vi "Select.vi"(8 "error in (no error)":errorcluster, 10 "State":string(combo), 11 "Reference Cluster":T1) -> (0 "error out":errorcluster, 2 "Count error?":bool, 3 "Confirmed?":bool)   [LabVIEW 2019, in "ZenGage v3.0 UI.lvclass"]
uses:
  ZenGage v3.0 UI.lvclass
panel:
  out "Verification":bool
  in  "Change":bool
  in  "Confirm":bool
  in  "OK Button":bool
  in  "Reset Button":bool
  in  "Total Count":string
  in  "Reel Count":string
  in  "Operator ID":string
  in  "Part Name":string(combo)
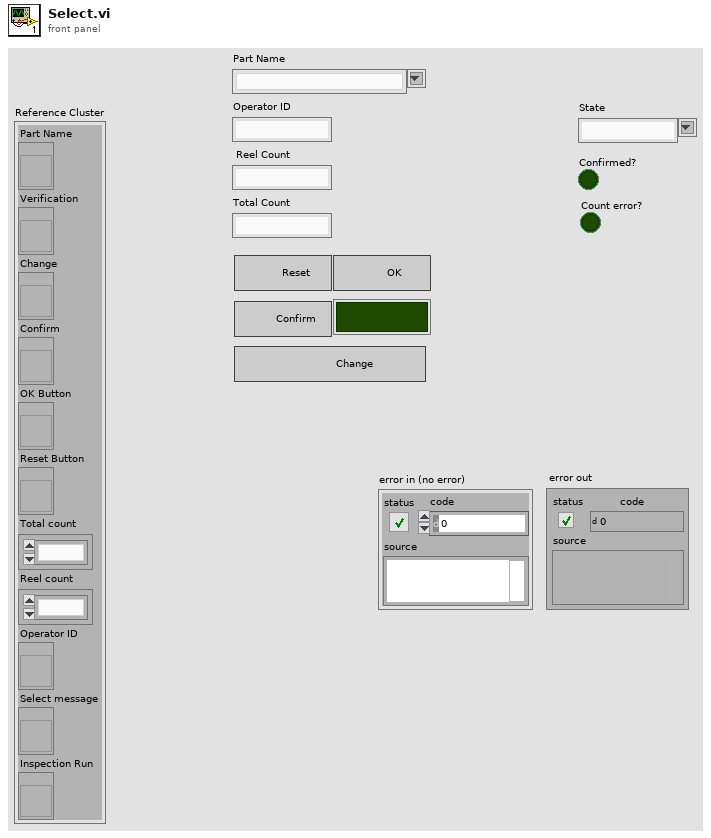
[diagram p1: front panel]
types:
  T1 = cluster{"Part Name":refnum<vi>, "Verification":refnum<vi>, "Change":refnum<vi>, "Confirm":refnum<vi>, "OK Button":refnum<vi>, "Reset Button":refnum<vi>, "Total count":refnum<vi>, "Reel count":refnum<vi>, "Operator ID":refnum<vi>, "Select message":refnum<vi>, "Inspection Run":refnum<vi>}
  T2 = enum8{"Enabled", "Disabled", "Disabled and Grayed Out"}
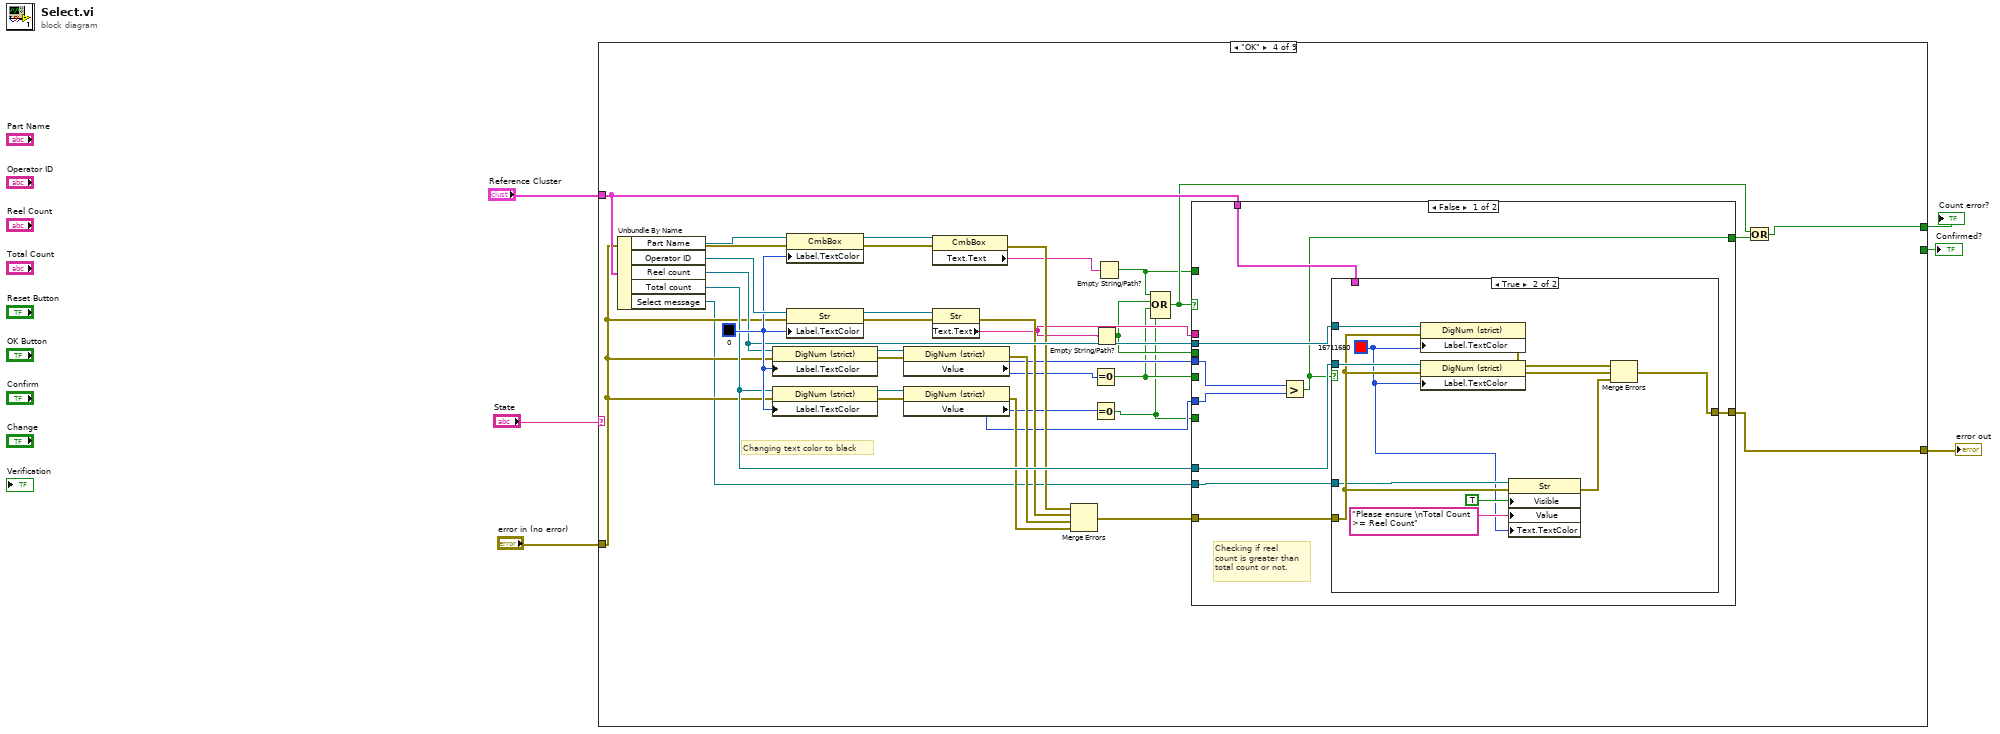
[diagram p0: block diagram]
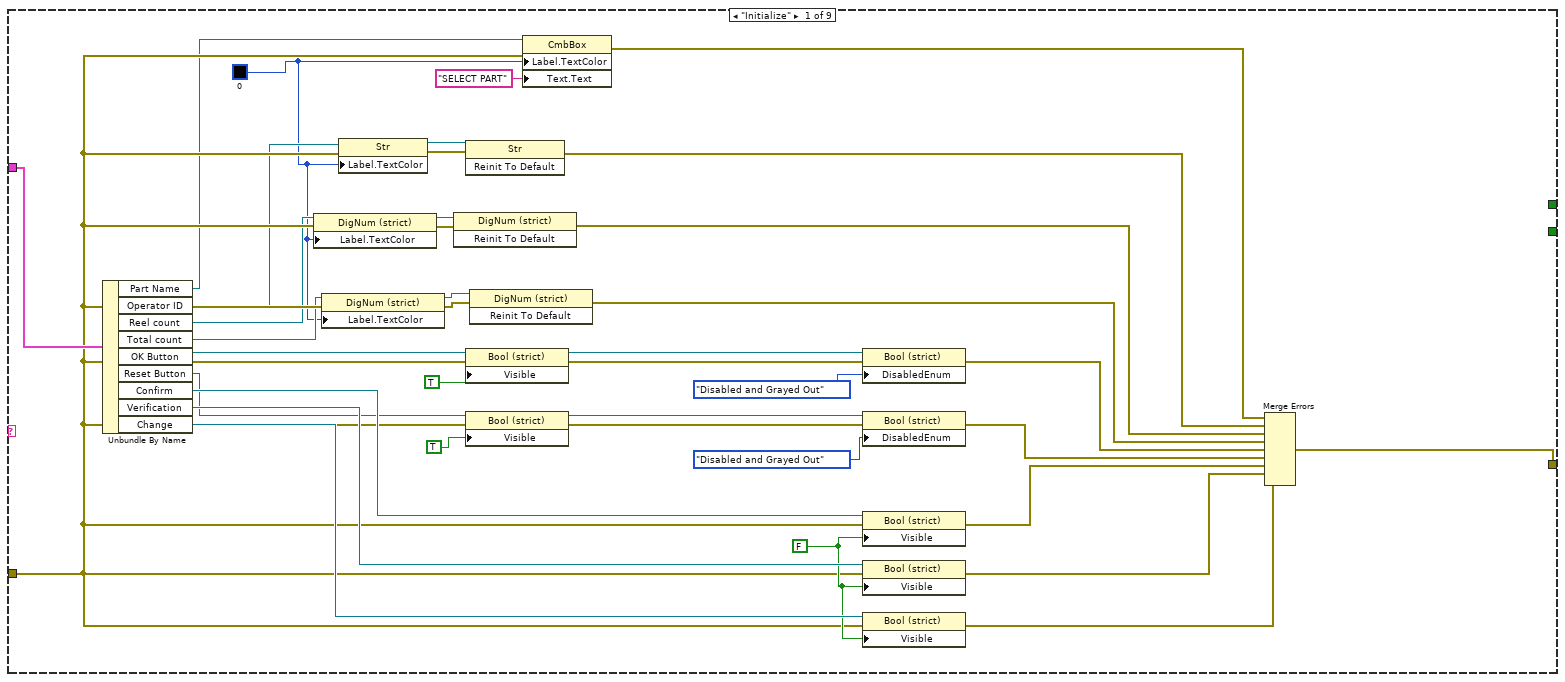
[diagram p2: hidden frame]
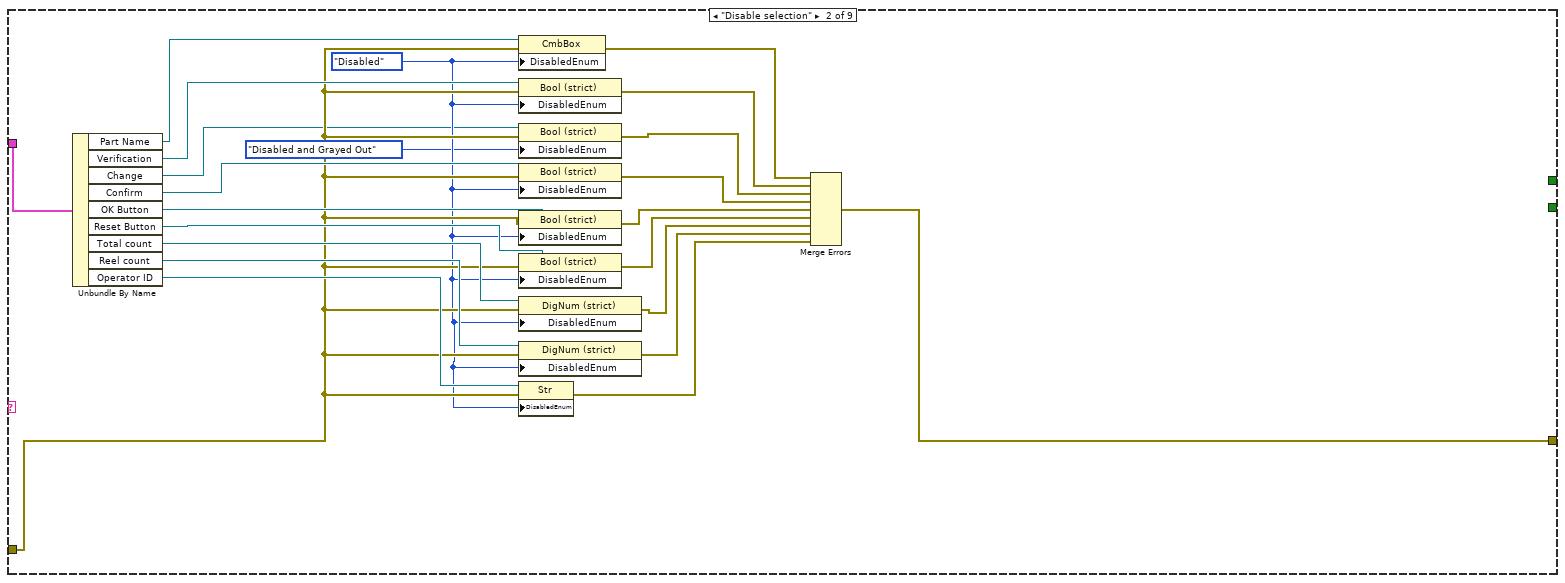
[diagram p3: hidden frame]
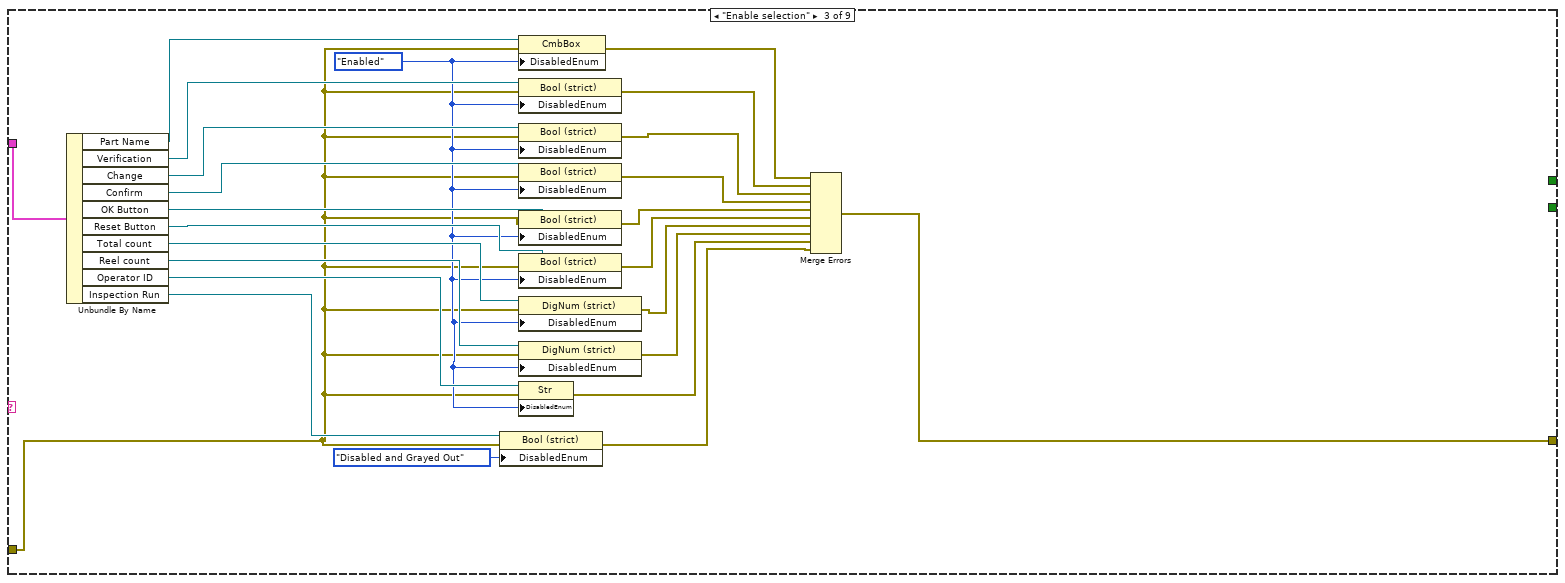
[diagram p4: hidden frame]
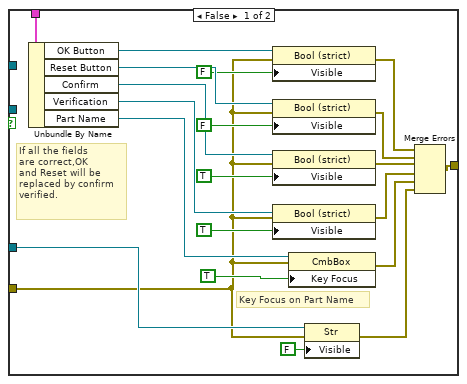
[diagram p5: hidden frame]
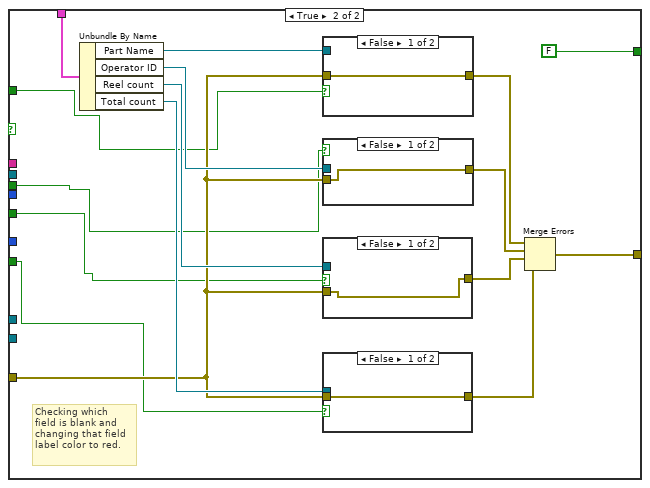
[diagram p6: hidden frame]
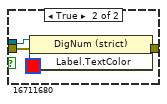
[diagram p7: hidden frame]
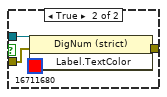
[diagram p8: hidden frame]
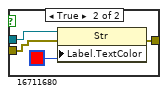
[diagram p9: hidden frame]
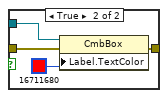
[diagram p10: hidden frame]
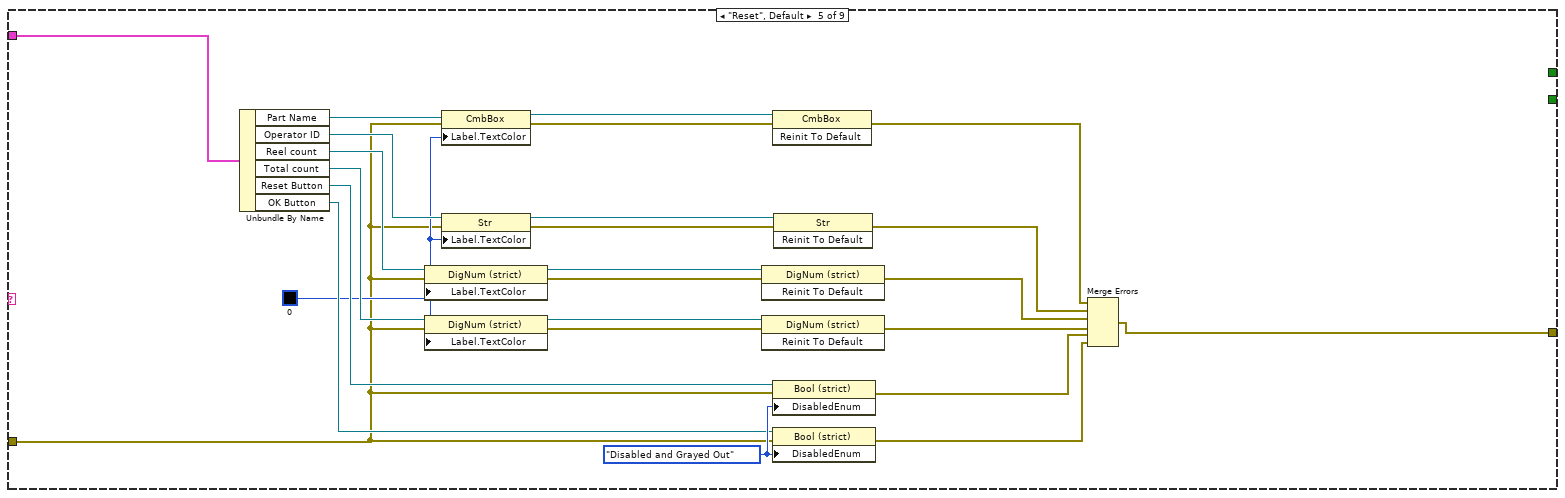
[diagram p11: hidden frame]
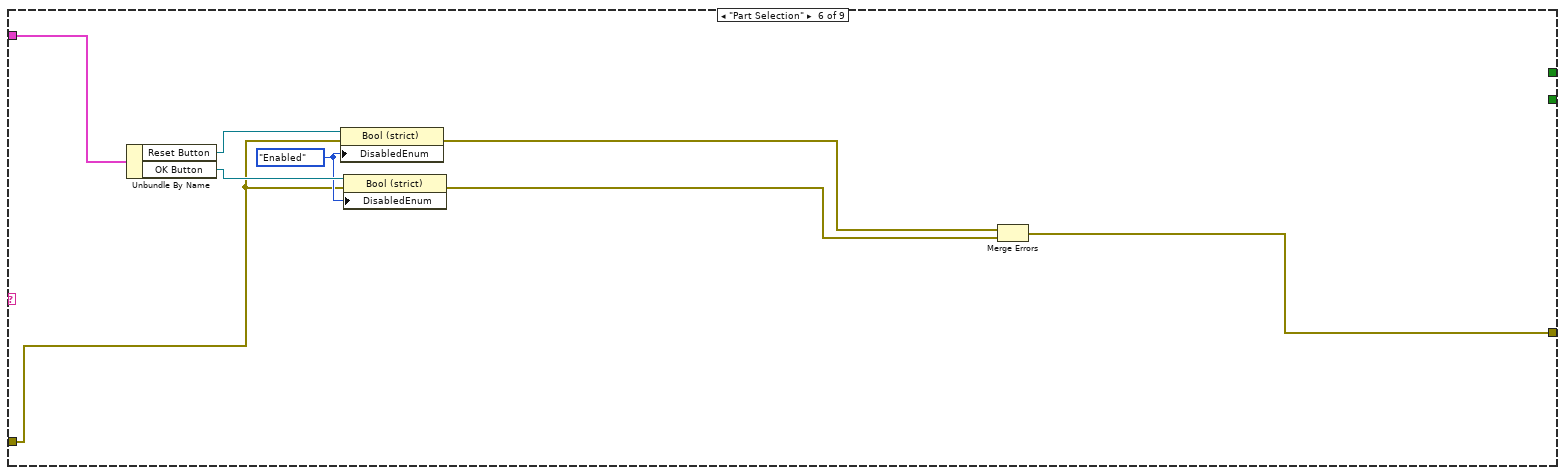
[diagram p12: hidden frame]
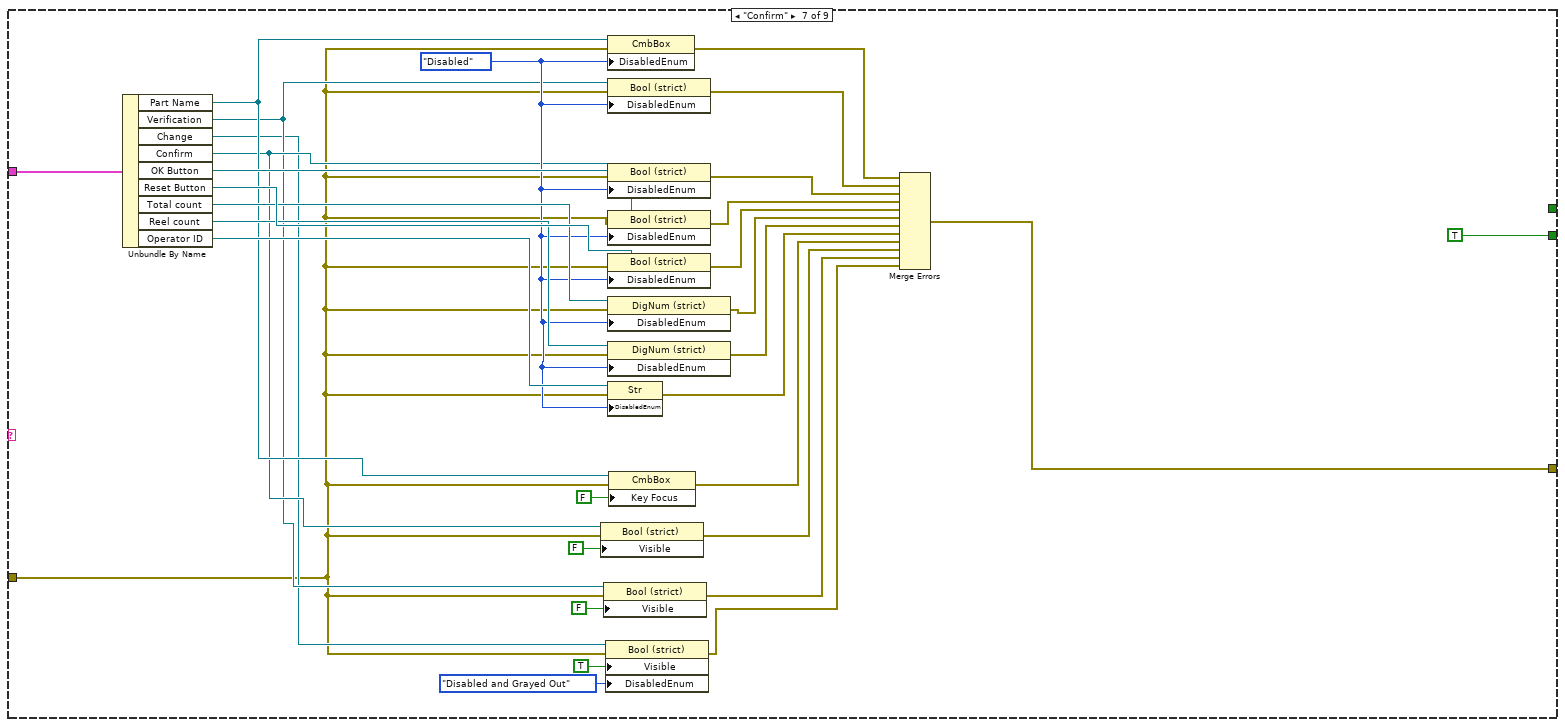
[diagram p13: hidden frame]
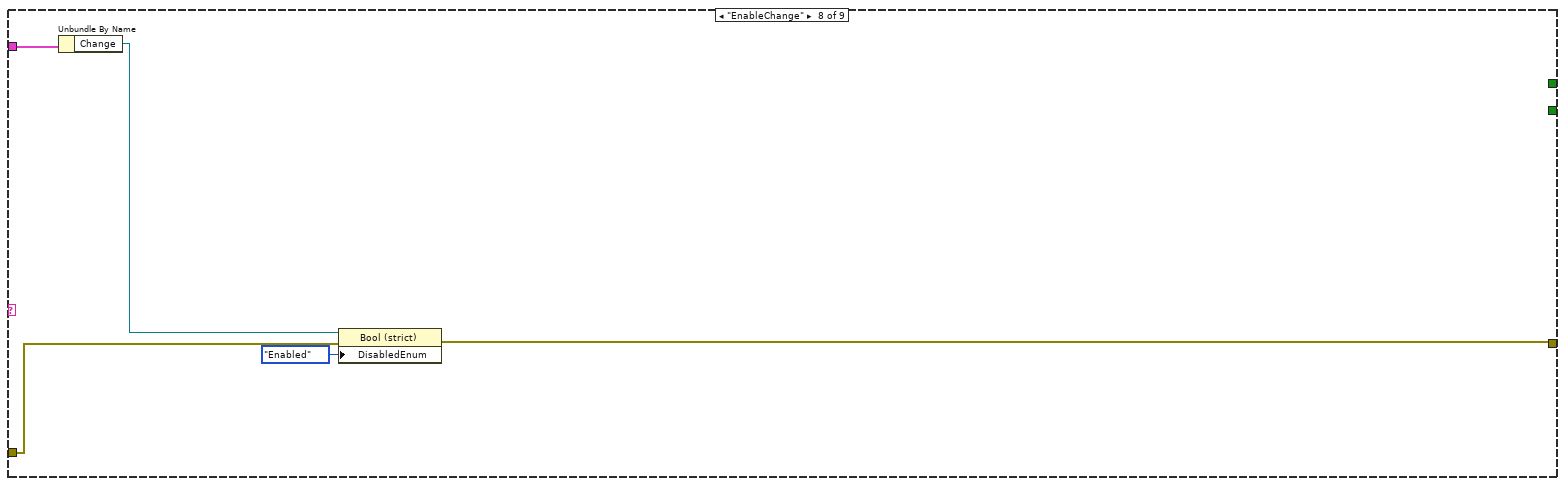
[diagram p14: hidden frame]
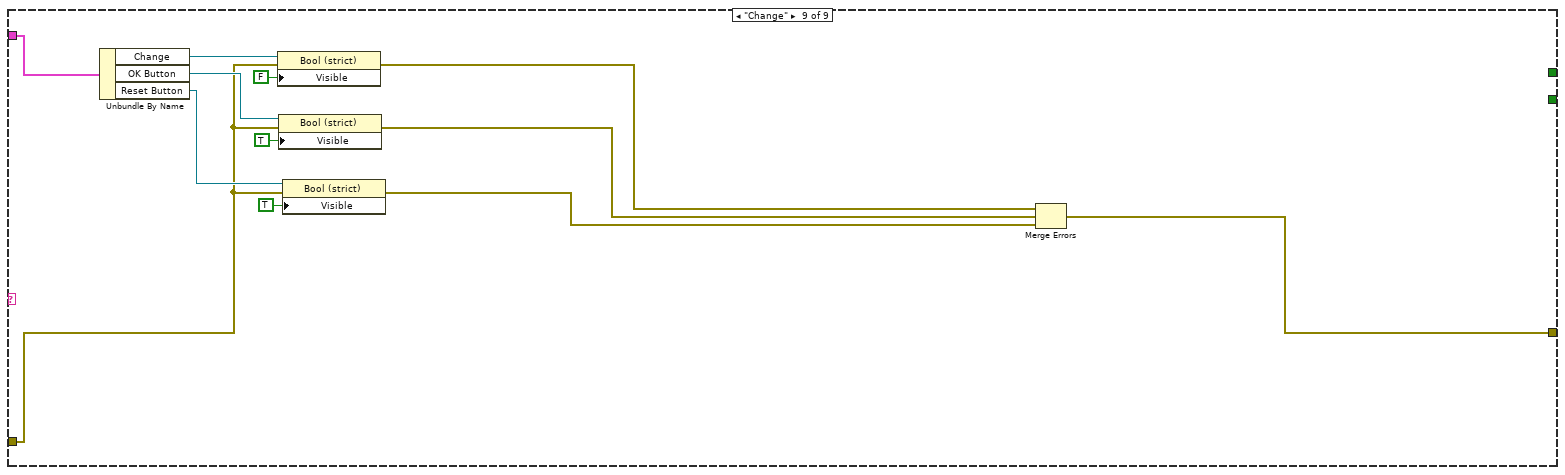
[diagram p15: hidden frame]
diagram:
  n1 = case shown="\"OK\"" "State" {
    tunnel: "Reference Cluster" -> [w42 w67 w92 w116 w219 w232 w243 w271 w283]
    tunnel: "error in (no error)" -> [w18 w49 w69 w115 w204 w228 w242 w270 w276]
    tunnel: [w32 w48 w73 w105 w203 w229 w237 w269 w272] -> w3
    tunnel: [_ _ _ _ _ _ TRUE _ _] -> w2
    tunnel: [_ _ _ w98 _ _ _ _ _] -> w1
    frame "Initialize" {
      w9 = u32 0
      w38 = FALSE ("Visible")
      n2 = Unbundle By Name(w42) -> ("Part Name"=w10:refnum<vi>, "Operator ID"=w16:refnum<vi>, "Reel count"=w14:refnum<vi>, "Total count"=w12:refnum<vi>, "OK Button"=w26:refnum<vi>, "Reset Button"=w24:refnum<vi>, "Confirm"=w41:refnum<vi>, "Verification"=w40:refnum<vi>, "Change"=w39:refnum<vi>)
      n3 = property class="DigNum (strict)"(reference=w14, error in=w18, "Label.TextColor"=w9) -> (reference out=w13:refnum<vi>, error out=w19:errorcluster)
      n4 = property class="DigNum (strict)"(reference=w12, error in=w18, "Label.TextColor"=w9) -> (reference out=w11:refnum<vi>, error out=w17:errorcluster)
      n5 = property class="Str"(reference=w16, error in=w18, "Label.TextColor"=w9) -> (reference out=w15:refnum<vi>, error out=w20:errorcluster)
      n6 = invoke class="DigNum (strict)" method="Reinit To Default"(reference=w13, error in=w19) -> (error out=w22:errorcluster)  [unwired: 1 in, 2 out]
      n7 = invoke class="Str" method="Reinit To Default"(reference=w15, error in=w20) -> (error out=w23:errorcluster)  [unwired: 1 in, 2 out]
      n8 = property class="Bool (strict)"(reference=w26, error in=w18, "Visible"=TRUE ("Value")) -> (reference out=w27:refnum<vi>, error out=w28:errorcluster)
      n9 = property class="Bool (strict)"(reference=w24, error in=w18, "Visible"=TRUE) -> (reference out=w31:refnum<vi>, error out=w30:errorcluster)
      n10 = invoke class="DigNum (strict)" method="Reinit To Default"(reference=w11, error in=w17) -> (error out=w21:errorcluster)  [unwired: 1 in, 2 out]
      n11 = property class="CmbBox"(reference=w10, error in=w18, "Label.TextColor"=w9, "Text.Text"="SELECT PART") -> (error out=w8:errorcluster)  [unwired: 1 out]
      n12 = property class="Bool (strict)"(reference=w27, error in=w28, "DisabledEnum"=T2."Disabled and Grayed Out" ("Disabled")) -> (error out=w37:errorcluster)  [unwired: 1 out]
      n13 = property class="Bool (strict)"(reference=w31, error in=w30, "DisabledEnum"=T2."Disabled and Grayed Out" ("Disabled")) -> (error out=w36:errorcluster)  [unwired: 1 out]
      n14 = property class="Bool (strict)"(reference=w41, error in=w18, "Visible"=w38) -> (error out=w35:errorcluster)  [unwired: 1 out]
      n15 = property class="Bool (strict)"(reference=w40, error in=w18, "Visible"=w38) -> (error out=w34:errorcluster)  [unwired: 1 out]
      n16 = property class="Bool (strict)"(reference=w39, error in=w18, "Visible"=w38) -> (error out=w33:errorcluster)  [unwired: 1 out]
      n17 = Merge Errors(w8, w23, w22, w21, w37, w36, w35, w34, w33) -> (w32:errorcluster)
    }
    frame "Disable selection" {
      w47 = T2."Disabled" ("Disabled")
      n18 = Unbundle By Name(w67) -> ("Part Name"=w66:refnum<vi>, "Verification"=w65:refnum<vi>, "Change"=w45:refnum<vi>, "Confirm"=w64:refnum<vi>, "OK Button"=w63:refnum<vi>, "Reset Button"=w62:refnum<vi>, "Total count"=w61:refnum<vi>, "Reel count"=w60:refnum<vi>, "Operator ID"=w59:refnum<vi>)
      n19 = property class="CmbBox"(reference=w66, error in=w49, "DisabledEnum"=w47) -> (error out=w58:errorcluster)  [unwired: 1 out]
      n20 = property class="Bool (strict)"(reference=w65, error in=w49, "DisabledEnum"=w47) -> (error out=w57:errorcluster)  [unwired: 1 out]
      n21 = property class="Bool (strict)"(reference=w45, error in=w49, "DisabledEnum"=T2."Disabled and Grayed Out" ("Disabled")) -> (error out=w56:errorcluster)  [unwired: 1 out]
      n22 = property class="Bool (strict)"(reference=w64, error in=w49, "DisabledEnum"=w47) -> (error out=w55:errorcluster)  [unwired: 1 out]
      n23 = property class="Bool (strict)"(reference=w63, error in=w49, "DisabledEnum"=w47) -> (error out=w54:errorcluster)  [unwired: 1 out]
      n24 = property class="Bool (strict)"(reference=w62, error in=w49, "DisabledEnum"=w47) -> (error out=w53:errorcluster)  [unwired: 1 out]
      n25 = property class="DigNum (strict)"(reference=w61, error in=w49, "DisabledEnum"=w47) -> (error out=w52:errorcluster)  [unwired: 1 out]
      n26 = property class="DigNum (strict)"(reference=w60, error in=w49, "DisabledEnum"=w47) -> (error out=w51:errorcluster)  [unwired: 1 out]
      n27 = property class="Str"(reference=w59, error in=w49, "DisabledEnum"=w47) -> (error out=w50:errorcluster)  [unwired: 1 out]
      n28 = Merge Errors(w58, w57, w56, w55, w54, w53, w52, w51, w50) -> (w48:errorcluster)
    }
    frame "Enable selection" {
      w72 = T2."Enabled" ("Disabled")
      n29 = Unbundle By Name(w92) -> ("Part Name"=w91:refnum<vi>, "Verification"=w90:refnum<vi>, "Change"=w89:refnum<vi>, "Confirm"=w88:refnum<vi>, "OK Button"=w87:refnum<vi>, "Reset Button"=w86:refnum<vi>, "Total count"=w85:refnum<vi>, "Reel count"=w84:refnum<vi>, "Operator ID"=w83:refnum<vi>, "Inspection Run"=w71:refnum<vi>)
      n30 = property class="Bool (strict)"(reference=w71, error in=w69, "DisabledEnum"=T2."Disabled and Grayed Out" ("Disabled")) -> (error out=w68:errorcluster)  [unwired: 1 out]
      n31 = property class="CmbBox"(reference=w91, error in=w69, "DisabledEnum"=w72) -> (error out=w82:errorcluster)  [unwired: 1 out]
      n32 = property class="Bool (strict)"(reference=w90, error in=w69, "DisabledEnum"=w72) -> (error out=w81:errorcluster)  [unwired: 1 out]
      n33 = property class="Bool (strict)"(reference=w89, error in=w69, "DisabledEnum"=w72) -> (error out=w80:errorcluster)  [unwired: 1 out]
      n34 = property class="Bool (strict)"(reference=w88, error in=w69, "DisabledEnum"=w72) -> (error out=w79:errorcluster)  [unwired: 1 out]
      n35 = property class="Bool (strict)"(reference=w87, error in=w69, "DisabledEnum"=w72) -> (error out=w78:errorcluster)  [unwired: 1 out]
      n36 = property class="Bool (strict)"(reference=w86, error in=w69, "DisabledEnum"=w72) -> (error out=w77:errorcluster)  [unwired: 1 out]
      n37 = property class="DigNum (strict)"(reference=w85, error in=w69, "DisabledEnum"=w72) -> (error out=w76:errorcluster)  [unwired: 1 out]
      n38 = property class="DigNum (strict)"(reference=w84, error in=w69, "DisabledEnum"=w72) -> (error out=w75:errorcluster)  [unwired: 1 out]
      n39 = property class="Str"(reference=w83, error in=w69, "DisabledEnum"=w72) -> (error out=w74:errorcluster)  [unwired: 1 out]
      n40 = Merge Errors(w82, w81, w80, w79, w78, w77, w76, w75, w74, w68) -> (w73:errorcluster)
    }
    frame "OK" {
      w119 = u32 0
      # "Changing text color to black"
      n41 = Unbundle By Name(w116) -> ("Part Name"=w125:refnum<vi>, "Operator ID"=w124:refnum<vi>, "Reel count"=w118:refnum<vi>, "Total count"=w117:refnum<vi>, "Select message"=w93:refnum<vi>)
      n42 = property class="DigNum (strict)"(reference=w118, error in=w115, "Label.TextColor"=w119) -> (reference out=w121:refnum<vi>, error out=w112:errorcluster)
      n43 = property class="DigNum (strict)"(reference=w117, error in=w115, "Label.TextColor"=w119) -> (reference out=w120:refnum<vi>, error out=w111:errorcluster)
      n44 = property class="CmbBox"(reference=w125, error in=w115, "Label.TextColor"=w119) -> (reference out=w123:refnum<vi>, error out=w114:errorcluster)
      n45 = property class="Str"(reference=w124, error in=w115, "Label.TextColor"=w119) -> (reference out=w122:refnum<vi>, error out=w113:errorcluster)
      n46 = property class="DigNum (strict)"(reference=w121, error in=w112) -> (error out=w108:errorcluster, "Value"=w102:u64)  [unwired: 1 out]
      n47 = property class="DigNum (strict)"(reference=w120, error in=w111) -> (error out=w107:errorcluster, "Value"=w101:u64)  [unwired: 1 out]
      n48 = property class="CmbBox"(reference=w123, error in=w114) -> (error out=w110:errorcluster, "Text.Text"=w104:string)  [unwired: 1 out]
      n49 = property class="Str"(reference=w122, error in=w113) -> (error out=w109:errorcluster, "Text.Text"=w103:string)  [unwired: 1 out]
      n50 = Merge Errors(w110, w109, w108, w107) -> (w106:errorcluster)
      n51 = Equal To 0?(x=w102) -> (x = 0?=w95:bool)
      n52 = Equal To 0?(x=w101) -> (x = 0?=w94:bool)
      n53 = Empty String/Path?(string/path=w103) -> (empty?=w96:bool)
      n54 = Empty String/Path?(string/path=w104) -> (empty?=w97:bool)
      n55 = Compound Arithmetic op=OR(w97, w96, w95, w94) -> (w99:bool)
      n56 = case shown="False" w99 {
        tunnel: w102 -> [w134 _]
        tunnel: w101 -> [w133 _]
        tunnel: w118 -> [w132 _]
        tunnel: w117 -> [w131 _]
        tunnel: w103 -> [_ _]
        tunnel: w116 -> [w130 w182]
        tunnel: w106 -> [w129 w177]
        tunnel: [w128 w172] -> w105
        tunnel: [w127 FALSE] -> w100
        tunnel: w97 -> [_ w170]
        tunnel: w96 -> [_ w169]
        tunnel: w95 -> [_ w168]
        tunnel: w94 -> [_ w167]
        tunnel: w93 -> [w126 _]
        frame False {
          # "Checking if reel\ncount is greater than\ntotal count or not."
          n57 = Greater?(x=w134, y=w133) -> (0:w127:bool)
          n58 = case shown="True" w127 {
            tunnel: w132 -> [_ w165]
            tunnel: w131 -> [_ w166]
            tunnel: w130 -> [w155 _]
            tunnel: w129 -> [w136 w161]
            tunnel: [w139 w162] -> w128
            tunnel: w126 -> [w138 w159]
            frame False {
              # "Key Focus on Part Name"
              # "If all the fields \nare correct,OK\nand Reset will be \nreplaced by confirm\nverified."
              n59 = Unbundle By Name(w155) -> ("OK Button"=w151:refnum<vi>, "Reset Button"=w152:refnum<vi>, "Confirm"=w153:refnum<vi>, "Verification"=w154:refnum<vi>, "Part Name"=w146:refnum<vi>)
              n60 = property class="Bool (strict)"(reference=w151, error in=w136, "Visible"=FALSE) -> (error out=w144:errorcluster)  [unwired: 1 out]
              n61 = property class="Bool (strict)"(reference=w152, error in=w136, "Visible"=FALSE) -> (error out=w143:errorcluster)  [unwired: 1 out]
              n62 = property class="Bool (strict)"(reference=w153, error in=w136, "Visible"=TRUE) -> (error out=w142:errorcluster)  [unwired: 1 out]
              n63 = property class="Bool (strict)"(reference=w154, error in=w136, "Visible"=TRUE) -> (error out=w141:errorcluster)  [unwired: 1 out]
              n64 = property class="CmbBox"(reference=w146, error in=w136, "Key Focus"=TRUE ("Visible")) -> (error out=w140:errorcluster)  [unwired: 1 out]
              n65 = property class="Str"(reference=w138, error in=w136, "Visible"=FALSE) -> (error out=w135:errorcluster)  [unwired: 1 out]
              n66 = Merge Errors(w144, w143, w142, w141, w140, w135) -> (w139:errorcluster)
            }
            frame True {
              w156 = u32 16711680
              n67 = property class="DigNum (strict)"(reference=w165, error in=w161, "Label.TextColor"=w156) -> (error out=w164:errorcluster)  [unwired: 1 out]
              n68 = property class="DigNum (strict)"(reference=w166, error in=w161, "Label.TextColor"=w156) -> (error out=w163:errorcluster)  [unwired: 1 out]
              n69 = property class="Str"(reference=w159, error in=w161, "Visible"=TRUE, "Value"="Please ensure \nTotal Count >= Reel Count", "Text.TextColor"=w156) -> (error out=w160:errorcluster)  [unwired: 1 out]
              n70 = Merge Errors(w164, w163, w160) -> (w162:errorcluster)
            }
          }
        }
        frame True {
          # "Checking which \nfield is blank and\nchanging that field\nlabel color to red."
          n71 = Unbundle By Name(w182) -> ("Part Name"=w181:refnum<vi>, "Operator ID"=w180:refnum<vi>, "Reel count"=w179:refnum<vi>, "Total count"=w178:refnum<vi>)
          n72 = case shown="False" w170 {
            tunnel: w181 -> [_ w201]
            tunnel: w177 -> [w198 w200]
            tunnel: [w198 w199] -> w176
            frame False {
            }
            frame True {
              n73 = property class="CmbBox"(reference=w201, error in=w200, "Label.TextColor"=u32 16711680) -> (error out=w199:errorcluster)  [unwired: 1 out]
            }
          }
          n74 = case shown="False" w169 {
            tunnel: w180 -> [_ w196]
            tunnel: w177 -> [w193 w195]
            tunnel: [w193 w194] -> w175
            frame False {
            }
            frame True {
              n75 = property class="Str"(reference=w196, error in=w195, "Label.TextColor"=u32 16711680) -> (error out=w194:errorcluster)  [unwired: 1 out]
            }
          }
          n76 = case shown="False" w168 {
            tunnel: w179 -> [_ w191]
            tunnel: w177 -> [w188 w190]
            tunnel: [w188 w189] -> w174
            frame False {
            }
            frame True {
              n77 = property class="DigNum (strict)"(reference=w191, error in=w190, "Label.TextColor"=u32 16711680) -> (error out=w189:errorcluster)  [unwired: 1 out]
            }
          }
          n78 = case shown="False" w167 {
            tunnel: w178 -> [_ w186]
            tunnel: w177 -> [w183 w185]
            tunnel: [w183 w184] -> w173
            frame False {
            }
            frame True {
              n79 = property class="DigNum (strict)"(reference=w186, error in=w185, "Label.TextColor"=u32 16711680) -> (error out=w184:errorcluster)  [unwired: 1 out]
            }
          }
          n80 = Merge Errors(w176, w175, w174, w173) -> (w172:errorcluster)
        }
      }
      n81 = Or(x=w99, y=w100) -> (x .or. y?=w98:bool)
    }
    frame "Reset", Default {
      w220 = u32 0
      w227 = T2."Disabled and Grayed Out" ("Disabled")
      n82 = Unbundle By Name(w219) -> ("Part Name"=w226:refnum<vi>, "Operator ID"=w225:refnum<vi>, "Reel count"=w224:refnum<vi>, "Total count"=w223:refnum<vi>, "Reset Button"=w222:refnum<vi>, "OK Button"=w221:refnum<vi>)
      n83 = property class="DigNum (strict)"(reference=w224, error in=w204, "Label.TextColor"=w220) -> (reference out=w216:refnum<vi>, error out=w212:errorcluster)
      n84 = property class="DigNum (strict)"(reference=w223, error in=w204, "Label.TextColor"=w220) -> (reference out=w215:refnum<vi>, error out=w211:errorcluster)
      n85 = property class="CmbBox"(reference=w226, error in=w204, "Label.TextColor"=w220) -> (reference out=w218:refnum<vi>, error out=w214:errorcluster)
      n86 = property class="Str"(reference=w225, error in=w204, "Label.TextColor"=w220) -> (reference out=w217:refnum<vi>, error out=w213:errorcluster)
      n87 = invoke class="DigNum (strict)" method="Reinit To Default"(reference=w216, error in=w212) -> (error out=w208:errorcluster)  [unwired: 1 in, 2 out]
      n88 = invoke class="DigNum (strict)" method="Reinit To Default"(reference=w215, error in=w211) -> (error out=w207:errorcluster)  [unwired: 1 in, 2 out]
      n89 = invoke class="CmbBox" method="Reinit To Default"(reference=w218, error in=w214) -> (error out=w210:errorcluster)  [unwired: 1 in, 2 out]
      n90 = property class="Bool (strict)"(reference=w222, error in=w204, "DisabledEnum"=w227) -> (error out=w206:errorcluster)  [unwired: 1 out]
      n91 = property class="Bool (strict)"(reference=w221, error in=w204, "DisabledEnum"=w227) -> (error out=w205:errorcluster)  [unwired: 1 out]
      n92 = invoke class="Str" method="Reinit To Default"(reference=w217, error in=w213) -> (error out=w209:errorcluster)  [unwired: 1 in, 2 out]
      n93 = Merge Errors(w210, w209, w208, w207, w206, w205) -> (w203:errorcluster)
    }
    frame "Part Selection" {
      w233 = T2."Enabled" ("Disabled")
      n94 = Unbundle By Name(w232) -> ("Reset Button"=w235:refnum<vi>, "OK Button"=w234:refnum<vi>)
      n95 = property class="Bool (strict)"(reference=w235, error in=w228, "DisabledEnum"=w233) -> (error out=w231:errorcluster)  [unwired: 1 out]
      n96 = property class="Bool (strict)"(reference=w234, error in=w228, "DisabledEnum"=w233) -> (error out=w230:errorcluster)  [unwired: 1 out]
      n97 = Merge Errors(w231, w230) -> (w229:errorcluster)
    }
    frame "Confirm" {
      w248 = T2."Disabled" ("Disabled")
      n98 = Unbundle By Name(w243) -> ("Part Name"=w247:refnum<vi>, "Verification"=w245:refnum<vi>, "Change"=w244:refnum<vi>, "Confirm"=w246:refnum<vi>, "OK Button"=w261:refnum<vi>, "Reset Button"=w260:refnum<vi>, "Total count"=w259:refnum<vi>, "Reel count"=w258:refnum<vi>, "Operator ID"=w257:refnum<vi>)
      n99 = property class="Bool (strict)"(reference=w246, error in=w242, "Visible"=FALSE) -> (error out=w240:errorcluster)  [unwired: 1 out]
      n100 = property class="Bool (strict)"(reference=w245, error in=w242, "Visible"=FALSE) -> (error out=w239:errorcluster)  [unwired: 1 out]
      n101 = property class="Bool (strict)"(reference=w244, error in=w242, "Visible"=TRUE, "DisabledEnum"=T2."Disabled and Grayed Out" ("Disabled")) -> (error out=w238:errorcluster)  [unwired: 1 out]
      n102 = property class="CmbBox"(reference=w247, error in=w242, "DisabledEnum"=w248) -> (error out=w256:errorcluster)  [unwired: 1 out]
      n103 = property class="Bool (strict)"(reference=w245, error in=w242, "DisabledEnum"=w248) -> (error out=w255:errorcluster)  [unwired: 1 out]
      n104 = property class="Bool (strict)"(reference=w246, error in=w242, "DisabledEnum"=w248) -> (error out=w254:errorcluster)  [unwired: 1 out]
      n105 = property class="Bool (strict)"(reference=w261, error in=w242, "DisabledEnum"=w248) -> (error out=w253:errorcluster)  [unwired: 1 out]
      n106 = property class="Bool (strict)"(reference=w260, error in=w242, "DisabledEnum"=w248) -> (error out=w252:errorcluster)  [unwired: 1 out]
      n107 = property class="DigNum (strict)"(reference=w259, error in=w242, "DisabledEnum"=w248) -> (error out=w251:errorcluster)  [unwired: 1 out]
      n108 = property class="DigNum (strict)"(reference=w258, error in=w242, "DisabledEnum"=w248) -> (error out=w250:errorcluster)  [unwired: 1 out]
      n109 = property class="Str"(reference=w257, error in=w242, "DisabledEnum"=w248) -> (error out=w249:errorcluster)  [unwired: 1 out]
      n110 = property class="CmbBox"(reference=w247, error in=w242, "Key Focus"=FALSE) -> (error out=w241:errorcluster)  [unwired: 1 out]
      n111 = Merge Errors(w256, w255, w254, w253, w252, w251, w250, w249, w241, w240, w239, w238) -> (w237:errorcluster)
    }
    frame "EnableChange" {
      n112 = Unbundle By Name(w271) -> ("Change"=w268:refnum<vi>)
      n113 = property class="Bool (strict)"(reference=w268, error in=w270, "DisabledEnum"=T2."Enabled" ("Disabled")) -> (error out=w269:errorcluster)  [unwired: 1 out]
    }
    frame "Change" {
      n114 = Unbundle By Name(w283) -> ("Change"=w282:refnum<vi>, "OK Button"=w281:refnum<vi>, "Reset Button"=w280:refnum<vi>)
      n115 = property class="Bool (strict)"(reference=w282, error in=w276, "Visible"=FALSE) -> (error out=w275:errorcluster)  [unwired: 1 out]
      n116 = property class="Bool (strict)"(reference=w281, error in=w276, "Visible"=TRUE) -> (error out=w274:errorcluster)  [unwired: 1 out]
      n117 = property class="Bool (strict)"(reference=w280, error in=w276, "Visible"=TRUE) -> (error out=w273:errorcluster)  [unwired: 1 out]
      n118 = Merge Errors(w275, w274, w273) -> (w272:errorcluster)
    }
  }
  "error out" <- w3
  "Confirmed?" <- w2
  "Count error?" <- w1
